vi "maxint.vi"() -> ()   [LabVIEW 2020]
uses:
  <vilib>/userdefined/High Color/IMAQdx.ctl
  C:/Users/lenovo/source/repos/MSMQ_try/how/bin/Release/how.dll
  source/repos/MSMQ_try/how/bin/Release/how.dll
  C:/Users/lenovo/source/repos/MSMQ_try/Calculator/bin/Debug/Calculator.dll
  source/repos/MSMQ_try/Calculator/bin/Debug/Calculator.dll
  C:/Users/lenovo/source/repos/MSMQ_try/Pallete_maker/bin/Debug/Pallete_maker.dll
  source/repos/MSMQ_try/Pallete_maker/bin/Debug/Pallete_maker.dll
  C:/Users/lenovo/source/repos/MSMQ_try/MIrror_x64/bin/Debug/MIrror_x64.dll
  source/repos/MSMQ_try/MIrror_x64/bin/Debug/MIrror_x64.dll
  <vilib>/vision/driver/NI_Vision_Acquisition_Software.lvlib
  <resource>/objmgr/imaqdx.rc
  source/repos/cont2019/x64/Release/Image_processing.dll
panel:
  in  "relax":bool
  in  "milliseconds to wait":u32=100
  out "maxium":u8
  in  "log_data":i32=1
  in  "Exposure time":dbl=5000.0
  out "Waveform Chart":u8(graph)
  in  "amplitude_limit":dbl=0.1
  in  "phi_v":dbl
  in  "phi_g":dbl=1.6
  in  "phi_p":dbl=1.2
  in  "vel_limit":dbl=0.4
  in  "init_zero":bool
  out "Waveform Graph 2":dbl[](graph)
  in  "stop":bool
  in  "cam":bool
  out "mirror params":string
  in  "DM":bool
  out "Iterations":i32
  out "global_best_value":dbl
  out "Waveform Graph":dbl[](graph)
  out "Image":T1(plugin-control)
  in  "Session In":T2="cam2"
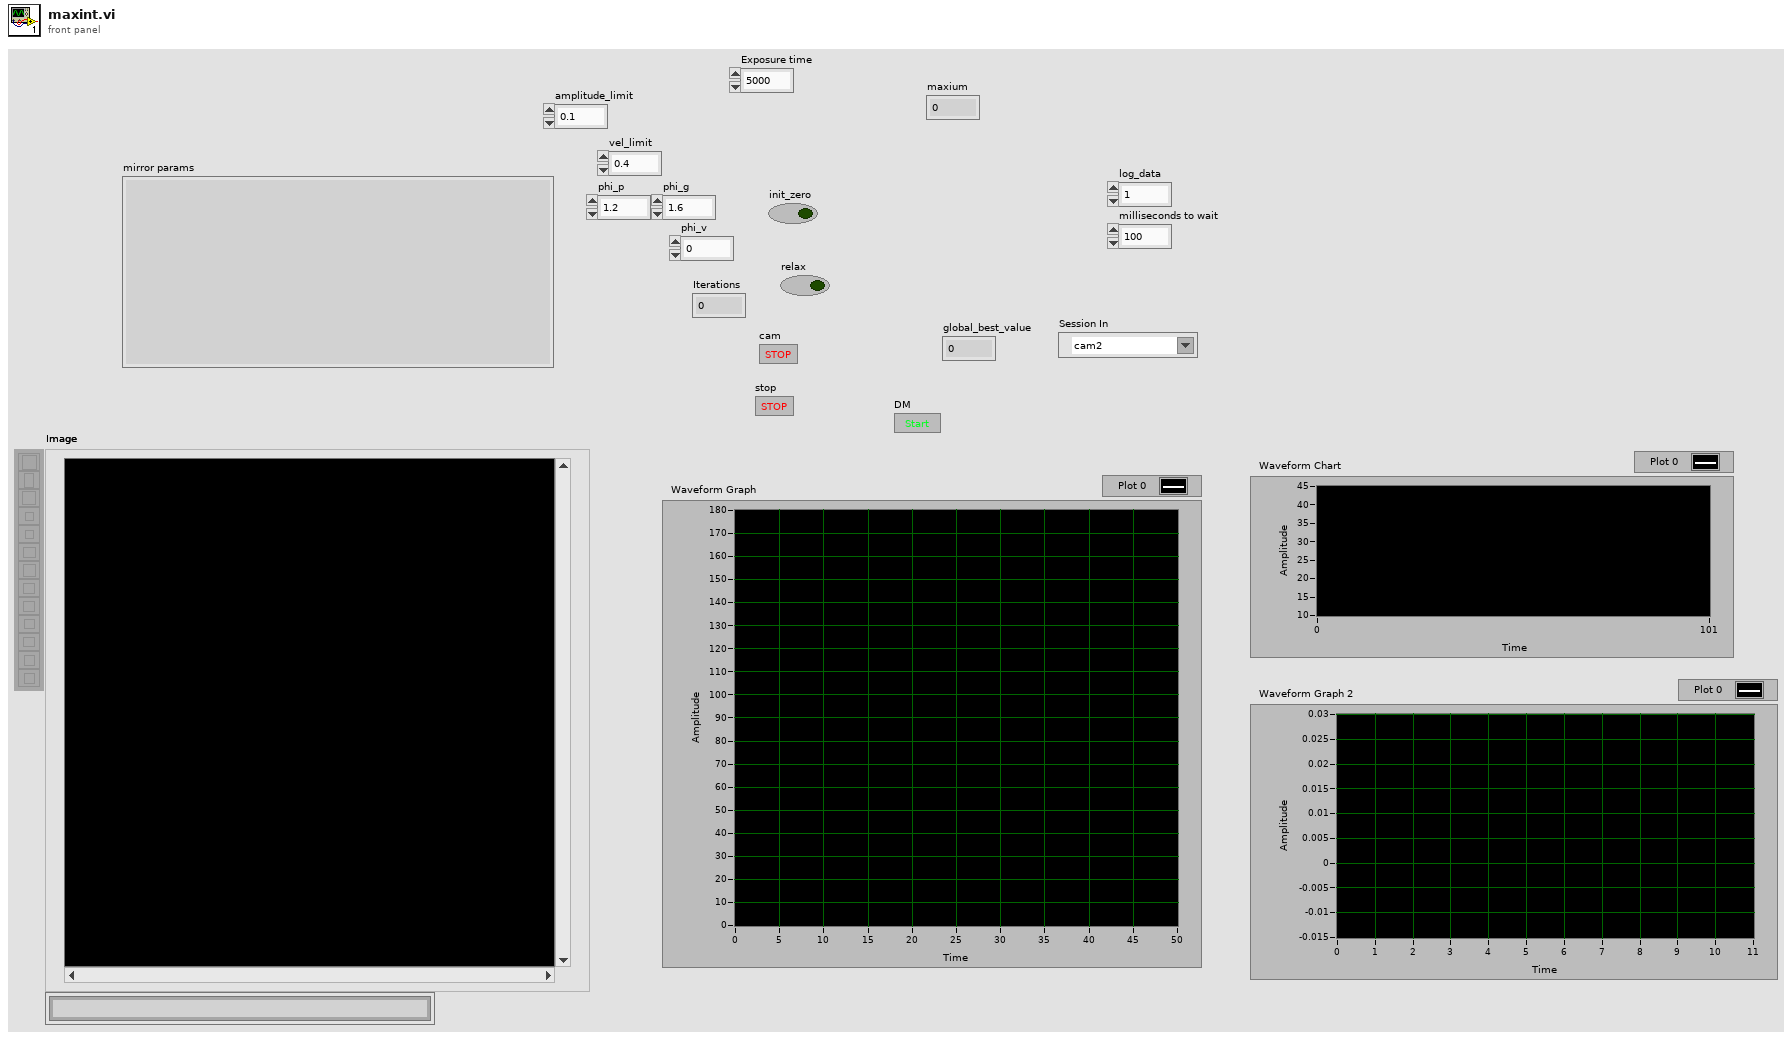
[diagram p1: front panel]
types:
  T1 = typedef "IMAQ Image.ctl" = refnum<image>
  T2 = typedef "IMAQdx.ctl" = refnum<k21>
  T3 = enum32{"Gray", "Binary", "Gradient", "Rainbow", "Temperature"}
  T4 = cluster{"Global Rectangle":i32[], "Contours":cluster{"Contour Type":u32, "ROI Type":u32, "Points":i32[]}[]}
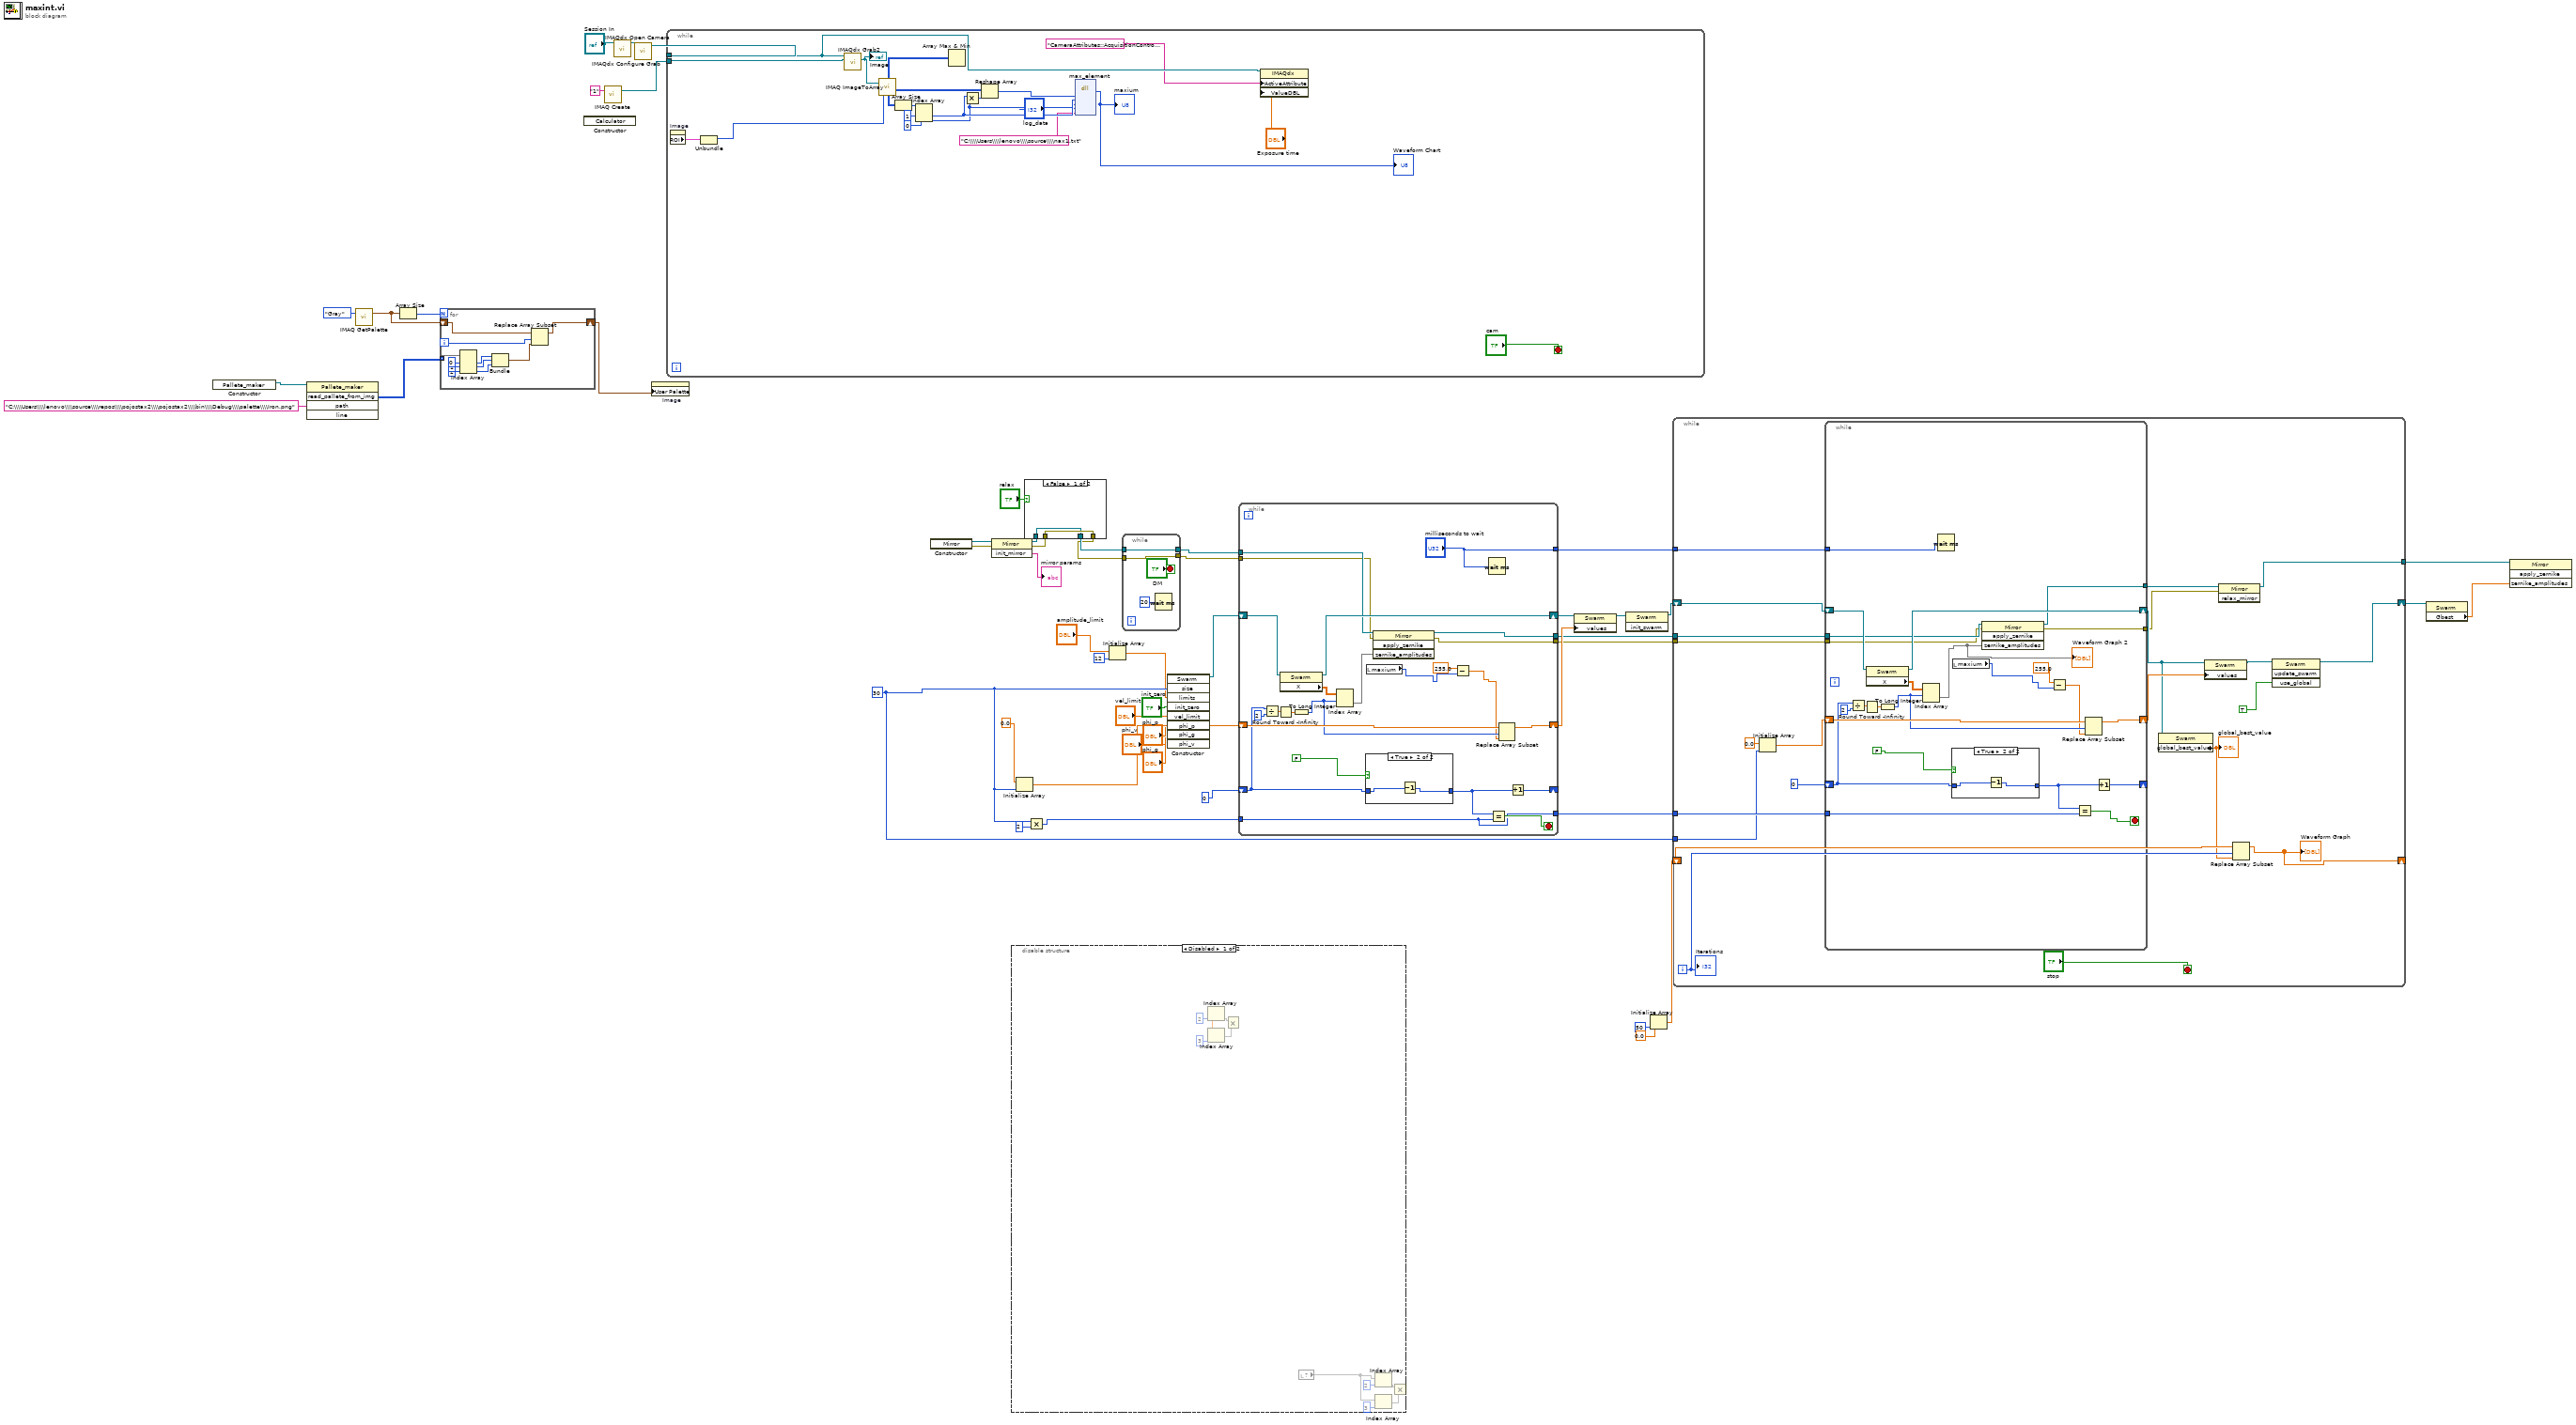
[diagram p0: block diagram]
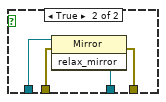
[diagram p2: hidden frame]
diagram:
  w28 = 30 ("size")
  n1 = constructor class="Pallete_maker"() -> (reference out=w41:refnum<k24>)  [unwired: 3 in, 2 out]
  n2 = invoke class="Pallete_maker" method="read_pallete_from_img"(reference=w41, "path"="C:\\\\Users\\\\lenovo\\\\source\\\\repos\\\\pojostax2\\\\pojostax2\\\\bin\\\\Debug\\\\palette\\\\Iron.png") -> ("read_pallete_from_img"=w42:u8[][])  [unwired: 3 in, 4 out]
  n3 = call "IMAQ GetPalette"("Palette Number (gray)"=T3."Gray") -> ("Color Palette"=w44:cluster{"Red":u8, "Green":u8, "Blue":u8}[])  [unwired: 4 in, 1 out]
  n4 = Array Size(array=w44) -> (size(s)=w45:i32)
  n5 = for {
    N: w45 -> [_]
    shift-right: [w52] -> w40
    shift-left: w44 -> [w54]
    tunnel: w42 -> [w62] mode=indexing
    i -> [w53]
    n6 = Index Array(array=w62, index #1=0 ("index"), index #2=1 ("index"), index #3=2 ("index")) -> (element #1=w58:u8, element #2=w57:u8, element #3=w56:u8)
    n7 = Bundle(w58, w57, w56) -> (w55:cluster{u8, u8, u8})  [unwired: 1 in]
    n8 = Replace Array Subset(array=w54, new element=w55, index=w53) -> (w52:cluster{"Red":u8, "Green":u8, "Blue":u8}[])
  }
  n9 = constructor class="Calculator"() -> ()  [unwired: 3 in, 3 out]
  n10 = call "IMAQ Create"("Image Name"="1") -> ("New Image"=w47:T1)  [unwired: 4 in, 1 out]
  n11 = call <vilib>:"IMAQdx Open Camera.vi"("Session In"="Session In") -> ("Session Out"=w49:T2)  [unwired: 9 in, 1 out]
  n12 = call <vilib>:"IMAQdx Configure Grab.vi"("Session In"=w49) -> ("Session Out"=w48:T2)  [unwired: 9 in, 1 out]
  n13 = property on="Image" class="ImageControl"("User Palette"=w40) -> ()  [unwired: 2 in, 2 out]
  n14 = while {
    tunnel: w48 -> [w70]
    tunnel: w47 -> [w81]
    stop <- "cam" stop-if-true
    n15 = property on="Image" class="ImageControl"() -> ("ROI"=w80:T4)  [unwired: 2 in, 2 out]
    n16 = Unbundle(w80) -> ("Global Rectangle"=w78:i32[])  [unwired: 1 out]
    n17 = call <vilib>:"IMAQdx Grab2.vi"("Image In"=w81, "Session In"=w70) -> ("Image Out"=w79:T1)  [unwired: 6 in, 3 out]
    "Image" <- w79
    n18 = call "IMAQ ImageToArray"("Optional Rectangle"=w78, "Image"=w79) -> ("Image Pixels (U8)"=w77:u8[][])  [unwired: 2 in, 4 out]
    n19 = Array Size(array=w77) -> (size(s)=w76:i32[])
    n20 = Index Array(array=w76, index #1=1 ("index"), index #2=0 ("index")) -> (element #1=w68:i32, element #2=w67:i32)
    n21 = Array Max & Min(array=w77) -> ()  [unwired: 4 out]
    n22 = Multiply(x=w68, y=w67) -> (x*y=w73:i32)
    n23 = Reshape Array(w77, w73) -> (w69:u8[])
    n24 = dll-call lib="C:/Users/lenovo/source/repos/cont2019/x64/Release/Image_processing.dll" fn="max_element"("pixel_data"=w69, "width"=w68, "height"=w67, "log_data"="log_data", "path"="C:\\\\Users\\\\lenovo\\\\source\\\\nax1.txt") -> ("maxium"=→"Waveform Chart" →"maxium":u8)  [unwired: 8 in, 2 out]
    n25 = property class="IMAQdx"(reference=w70, "ActiveAttribute"="CameraAttributes::AcquisitionControl::ExposureTime" ("ValueString"), "ValueDBL"="Exposure time") -> ()  [unwired: 1 in, 2 out]
  }
  n26 = constructor class="Mirror"() -> (reference out=w24:refnum<k24>, error out=w22:errorcluster)  [unwired: 3 in, 1 out]
  n27 = invoke class="Mirror" method="init_mirror"(reference=w24, error in=w22) -> (reference out=w17:refnum<k24>, error out=w16:errorcluster, "init_mirror"=→"mirror params":string)  [unwired: 1 in]
  n28 = disable-structure shown="Disabled" {
    frame Disabled {
      n29 = Index Array(index=3) -> (array=w82:dbl[], element=w86)
      n30 = Index Array(array=w82, index=2) -> (element=w85)
      n31 = Multiply(x=w85, y=w86) -> ()  [unwired: 1 out]
      n32 = local read item#-1() -> (w87)
      n33 = Index Array(array=w87, index=2) -> (element=w90)
      n34 = Index Array(array=w87, index=3) -> (element=w91)
      n35 = Multiply(x=w90, y=w91) -> ()  [unwired: 1 out]
    }
    frame Enabled {
    }
  }
  n36 = Initialize Array(0.0 ("element"), w28) -> (w36:dbl[])
  n37 = case shown="False" "relax" {
    tunnel: w17 -> [w92 w97]
    tunnel: w16 -> [w93 w96]
    tunnel: [w92 w95] -> w15
    tunnel: [w93 w94] -> w14
    frame False {
    }
    frame True {
      n38 = invoke class="Mirror" method="relax_mirror"(reference=w97, error in=w96) -> (reference out=w95:refnum<k24>, error out=w94:errorcluster)  [unwired: 1 in, 1 out]
    }
  }
  n39 = Multiply(x=w28, y=2) -> (x*y=w31:i32)
  n40 = Initialize Array("amplitude_limit", 12 ("dimension size")) -> (w6:dbl[])
  n41 = while {
    tunnel: [w100] -> w21
    tunnel: w15 -> [w100]
    tunnel: [w98] -> w20
    tunnel: w14 -> [w98]
    stop <- "DM" stop-if-true
    n42 = Wait (ms)(milliseconds to wait=u32 20) -> ()  [unwired: 1 out]
  }
  n43 = constructor class="Swarm"("size"=w28, "limits"=w6, "init_zero"="init_zero", "vel_limit"="vel_limit", "phi_p"="phi_p", "phi_g"="phi_g", "phi_v"="phi_v") -> (reference out=w37:refnum<k24>)  [unwired: 3 in, 9 out]
  n44 = while {
    shift-right: [w119] -> w34
    shift-left: w36 -> [w120]
    shift-right: [w117] -> w35
    shift-left: w37 -> [w125]
    shift-right: [w116] -> _
    shift-left: 0 -> [w114]
    tunnel: w31 -> [w112]
    tunnel: [w112] -> w29
    tunnel: w21 -> [w111]
    tunnel: w20 -> [w109]
    tunnel: [w108] -> w19
    tunnel: [w107] -> w18
    tunnel: ["milliseconds to wait"] -> w2
    stop <- w115 stop-if-true
    n45 = Divide(x=w114, y=2) -> (x/y=w123:dbl)
    n46 = Round Toward -Infinity(1:w123) -> (0:w122:dbl)
    n47 = property class="Swarm"(reference=w125) -> (reference out=w117:refnum<k24>, "X"=w121:dbl[][])  [unwired: 1 in, 1 out]
    n48 = To Long Integer(number=w122) -> (32bit integer=w118:i32)
    n49 = Index Array(array=w121, index (row)=w118) -> (element=w110:dbl[])  [unwired: 1 in]
    n50 = case shown="True" FALSE {
      tunnel: w114 -> [w126 w128]
      tunnel: [w126 w127] -> w113
      frame False {
      }
      frame True {
        n51 = Decrement(x=w128) -> (x-1=w127:i32)
      }
    }
    n52 = local read "maxium"() -> (w103:u8)
    n53 = invoke class="Mirror" method="apply_zernike"(reference=w111, error in=w109, "zernike_amplitudes"=w110) -> (reference out=w108:refnum<k24>, error out=w107:errorcluster)  [unwired: 1 in, 2 out]
    n54 = Subtract(x=255.0, y=w103) -> (x-y=w105:dbl)
    n55 = Wait (ms)(milliseconds to wait="milliseconds to wait") -> ()  [unwired: 1 out]
    n56 = Equal?(x=w113, y=w112) -> (x = y?=w115:bool)
    n57 = Replace Array Subset(array=w120, new element=w105, index=w118) -> (w119:dbl[])
    n58 = Increment(x=w113) -> (x+1=w116:i32)
  }
  n59 = property class="Swarm"(reference=w35, "values"=w34) -> (reference out=w33:refnum<k24>)  [unwired: 1 in, 1 out]
  n60 = invoke class="Swarm" method="init_swarm"(reference=w33) -> (reference out=w30:refnum<k24>)  [unwired: 2 in, 2 out]
  n61 = Initialize Array(0.0 ("element"), 50 ("dimension size")) -> (w25:dbl[])
  n62 = while {
    tunnel: w29 -> [w148]
    tunnel: w28 -> [w147]
    shift-right: [w141] -> w4
    shift-left: w30 -> [w150]
    shift-right: [w136] -> _
    shift-left: w25 -> [w139]
    tunnel: w19 -> [w135]
    tunnel: w18 -> [w134]
    tunnel: [w130] -> w5
    tunnel: w2 -> [w129]
    i -> [w138]
    stop <- "stop" stop-if-true
    n63 = Initialize Array(0.0 ("element"), w147) -> (w145:dbl[])
    n64 = while {
      shift-right: [w168] -> w144
      shift-left: w145 -> [w169]
      shift-right: [w166] -> w140
      shift-left: w150 -> [w174]
      shift-right: [w165] -> _
      shift-left: 0 -> [w163]
      tunnel: w148 -> [w164]
      tunnel: w135 -> [w161]
      tunnel: w134 -> [w160]
      tunnel: [w159] -> w133
      tunnel: [w158] -> w132
      tunnel: w129 -> [w151]
      stop <- w157 stop-if-true
      n65 = Divide(x=w163, y=2) -> (x/y=w172:dbl)
      n66 = Round Toward -Infinity(1:w172) -> (0:w171:dbl)
      n67 = property class="Swarm"(reference=w174) -> (reference out=w166:refnum<k24>, "X"=w170:dbl[][])  [unwired: 1 in, 1 out]
      n68 = To Long Integer(number=w171) -> (32bit integer=w167:i32)
      n69 = Index Array(array=w170, index (row)=w167) -> (element=w156:dbl[])  [unwired: 1 in]
      "Waveform Graph 2" <- w156
      n70 = Wait (ms)(milliseconds to wait=w151) -> ()  [unwired: 1 out]
      n71 = case shown="True" FALSE {
        tunnel: w163 -> [w175 w177]
        tunnel: [w175 w176] -> w162
        frame False {
        }
        frame True {
          n72 = Decrement(x=w177) -> (x-1=w176:i32)
        }
      }
      n73 = local read "maxium"() -> (w152:u8)
      n74 = invoke class="Mirror" method="apply_zernike"(reference=w161, error in=w160, "zernike_amplitudes"=w156) -> (reference out=w159:refnum<k24>, error out=w158:errorcluster)  [unwired: 1 in, 2 out]
      n75 = Subtract(x=255.0, y=w152) -> (x-y=w154:dbl)
      n76 = Equal?(x=w162, y=w164) -> (x = y?=w157:bool)
      n77 = Replace Array Subset(array=w169, new element=w154, index=w167) -> (w168:dbl[])
      n78 = Increment(x=w162) -> (x+1=w165:i32)
    }
    n79 = property class="Swarm"(reference=w140) -> ("global_best_value"=w137:dbl)  [unwired: 1 in, 2 out]
    "global_best_value" <- w137
    n80 = property class="Swarm"(reference=w140, "values"=w144) -> (reference out=w143:refnum<k24>)  [unwired: 1 in, 1 out]
    n81 = invoke class="Mirror" method="relax_mirror"(reference=w133, error in=w132) -> (reference out=w130:refnum<k24>)  [unwired: 1 in, 2 out]
    n82 = Replace Array Subset(array=w139, new element=w137, index=w138) -> (w136:dbl[])
    "Waveform Graph" <- w136
    n83 = invoke class="Swarm" method="update_swarm"(reference=w143, "use_global"=TRUE) -> (reference out=w141:refnum<k24>)  [unwired: 2 in, 3 out]
    "Iterations" <- w138
  }
  n84 = property class="Swarm"(reference=w4) -> ("Gbest"=w3:dbl[])  [unwired: 1 in, 2 out]
  n85 = invoke class="Mirror" method="apply_zernike"(reference=w5, "zernike_amplitudes"=w3) -> ()  [unwired: 2 in, 4 out]
